vi "LoopScript_EllipticOscillatory.vi"() -> ()   [LabVIEW 2017]
uses:
  CircleControls.ctl
  ImageAcquisitionProgram/ImageAcquisitionLibrary/GlobalFrontPanelReferences.vi
  AODControl/AODGlobals.vi
  AODControl/MessageQueue/QueueOperations/Enqueue Message (Single).vi
  ImageAcquisitionProgram/ImageAcquisitionLibrary/ImageAcquisitionLibrary.lvlib
  AODControl/AODControl.lvlib
  AODControl/MessageQueue/MessageQueue.lvlib
panel:
  in  "Run":bool
  out "Area":dbl
  out "Eccentricity":dbl
  out "Radius":dbl
  in  "Transform\nSeconds":i32=60
  in  "oscillation \nangle":dbl=0.03 format="%#_13g"
  in  "No. of Points":i32=33
  out "Total Running \nTime":dbl=90000.0 format="%<%H:%M:%S>t"
  in  "period (s)":dbl=1.0
  out "Area":dbl[](array[numeric])=[98.5203456165759, 93.52521329736813, 88.53008097816036, 83.5349486589526, 78.53981633974483]
  out "Radius":dbl[](array[numeric])=[5.6, 5.4561891462814955, 5.308483775994799, 5.156549233741495, 5.0]
  out "Eccentricity":dbl[](array[numeric])=[1.0, 1.25, 1.5, 1.75, 2.0]
  in  "e_0":dbl=1.0
  in  "e_f":dbl=2.0
  in  "Eccentricity \nSteps":i32=5
  in  "R_f":dbl=5.0
  in  "R_0":dbl=5.6
  in  "Packing Steps":i32=5
  in  "Number of \nPeriods":u32=3600
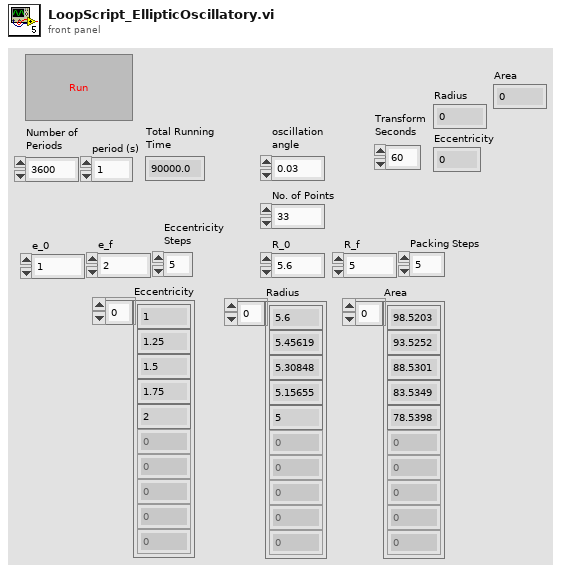
[diagram p1: front panel]
types:
  T1 = typedef "CircleControls.ctl" = cluster{"Radius":dbl, "No. of Points":i32, "Center":cluster{"X":dbl, "Y":dbl}, "Circle":bool, "Density":dbl, "PointSpec":enum32{"No. Of Points", "Density"}, "Hold":bool, "Size":i32, "LatC":dbl, "Eccentricity":dbl, "Phase":dbl}
  T2 = typedef "AODControl.lvlib/InterfaceReferences.ctl" = cluster{"AOD Points Display":refnum<vi>, "AOD Array":refnum<vi>, "AOD Array Size":refnum<vi>, "Replace Array List":refnum<vi>, "Replace List":refnum<vi>, "Remove":refnum<vi>, "Index":refnum<vi>, "Move":refnum<vi>, "X":refnum<vi>, "Y":refnum<vi>, "Add":refnum<vi>, "Load":refnum<vi>, "Save":refnum<vi>, "Exit":refnum<vi>, "Dynamic":refnum<vi>, "Rotate":refnum<vi>, "Rotation Speed":refnum<vi>, "Scaling Speed":refnum<vi>, "X Trans Speed":refnum<vi>, "Y Trans Speed":refnum<vi>, "Movie Array":refnum<vi>, "Play":refnum<vi>, "Playing Time":refnum<vi>}
  T3 = typedef "AODControl.lvlib/MessageQueue.lvlib/All Message Queues.ctl" = cluster{" AOD Interface":refnum<queue>}
  T4 = typedef "ImageAcquisitionLibrary.lvlib/References.ctl" = cluster{"Acquire":refnum<vi>, "Rec":refnum<vi>, "Tracking":refnum<vi>, "Settings":refnum<vi>, "Stop":refnum<vi>, "Initialized?":bool, "ImDisplay":refnum<vi>}
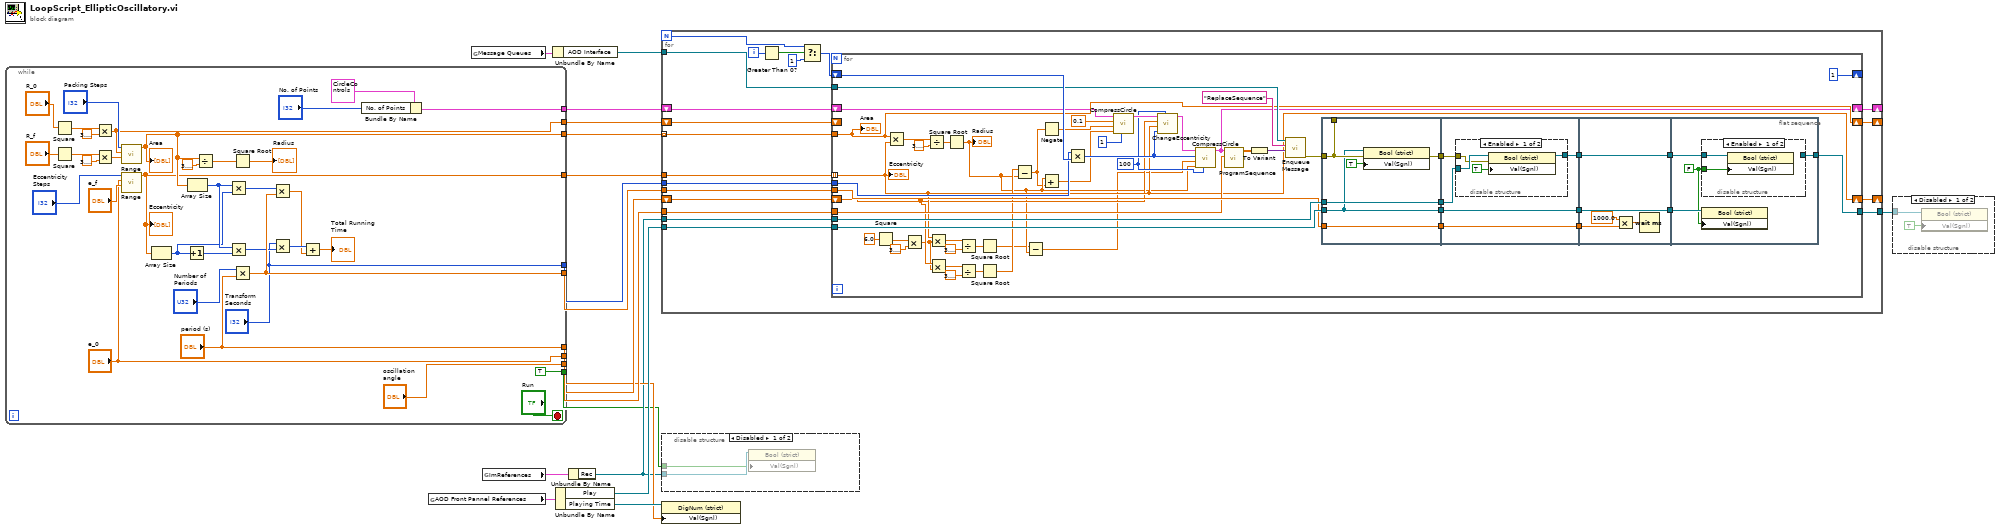
[diagram p0: block diagram]
diagram:
  n1 = while {
    tunnel: [w43] -> w18
    tunnel: [w39] -> w17
    tunnel: ["oscillation \nangle"] -> w16
    tunnel: [w35] -> w12
    tunnel: ["e_0"] -> w11
    tunnel: [w31] -> w10
    tunnel: [w30] -> w7
    tunnel: ["period (s)"] -> w5
    tunnel: ["Transform\nSeconds"] -> w4
    tunnel: [TRUE ("Value (Signaling)")] -> w1
    stop <- "Run" stop-if-true
    n2 = Square(x="R_0") -> (x^2=w51:dbl)
    n3 = Square(x="R_f") -> (x^2=w33:dbl)
    n4 = Multiply(x=w51, y=3.141592653589793) -> (x*y=w31:dbl)
    n5 = Multiply(x=w33, y=3.141592653589793) -> (x*y=w34:dbl)
    n6 = call "Range.vi"("End"=w34, "Start"=w31, "Steps"="Packing Steps") -> ("Array"=w43:dbl[])  [unwired: 8 in]
    "Area" <- w43
    n7 = call "Range.vi"("End"="e_f", "Start"="e_0", "Steps"="Eccentricity \nSteps") -> ("Array"=w35:dbl[])  [unwired: 8 in]
    "Eccentricity" <- w35
    n8 = Array Size(array=w35) -> (size(s)=w27:i32)
    n9 = Array Size(array=w43) -> (size(s)=w28:i32)
    n10 = Increment(x=w27) -> (x+1=w26:i32)
    n11 = Divide(x=w43, y=3.141592653589793) -> (x/y=w46:dbl[])
    n12 = Multiply(x=w28, y=w27) -> (x*y=w42:i32)
    n13 = Multiply(x=w28, y=w26) -> (x*y=w25:i32)
    n14 = Square Root(x=w46) -> (sqrt(x)=→"Radius":dbl[])
    n15 = Multiply(x="Number of \nPeriods", y="period (s)") -> (x*y=w30:dbl)
    n16 = Multiply(x=w42, y=w30) -> (x*y=w22:dbl)
    n17 = Multiply(x="Transform\nSeconds", y=w25) -> (x*y=w23:i32)
    n18 = Add(x=w23, y=w22) -> (x+y=→"Total Running \nTime":dbl)
    n19 = Bundle By Name(cluster=T1 {"Radius"=5.2, "No. of Points"=33, "Center"={"X"=0.0, "Y"=0.0}, "Circle"=TRUE, "Density"=1.0100217542370282, "PointSpec"=enum."No. Of Points", "Hold"=FALSE, "Size"=1, "LatC"=10.0, "Eccentricity"=1.0, "Phase"=0.0} ("Cluster"), "No. of Points"="No. of Points") -> (w39:T1)
  }
  n20 = global read "AODGlobals.vi" "AOD Front Pannel References"() -> (w9:T2)
  n21 = global read "AODGlobals.vi" "Message Queues"() -> (w14:T3)
  n22 = global read "GlobalFrontPanelReferences.vi" "ImReferences"() -> (w15:T4)
  n23 = Unbundle By Name(w14) -> ("AOD Interface"=w13:refnum<queue>)
  n24 = Unbundle By Name(w9) -> ("Play"=w8:refnum<vi>, "Playing Time"=w6:refnum<vi>)
  n25 = Unbundle By Name(w15) -> ("Rec"=w3:refnum<vi>)
  n26 = for {
    N -> [w58]
    tunnel: w18 -> [w67] mode=indexing
    tunnel: w12 -> [w56]
    tunnel: w16 -> [w73]
    tunnel: w13 -> [w72]
    tunnel: w4 -> [w71]
    shift-right: [w68] -> _
    shift-left: w10 -> [w66]
    shift-right: [w70] -> _
    shift-left: w11 -> [w69]
    tunnel: w8 -> [w65]
    tunnel: w3 -> [w64]
    tunnel: w7 -> [w63]
    tunnel: [w62] -> w2
    shift-right: [w55] -> _
    shift-left: w17 -> [w54]
    i -> [w61]
    n27 = Greater Than 0?(x=w61) -> (x > 0?=w60:bool)
    n28 = Select(t=w58, s=w60, f=1) -> (s? t:f=w57:i32)
    n29 = for {
      tunnel: w56 -> [w87] mode=indexing
      tunnel: w67 -> [w105]
      tunnel: w73 -> [w103]
      shift-right: [w105] -> w68
      shift-left: w66 -> [_]
      tunnel: w72 -> [w106]
      tunnel: w71 -> [w104]
      shift-right: [w87] -> w70
      shift-left: w69 -> [w80]
      tunnel: w65 -> [w122]
      tunnel: w64 -> [w119]
      tunnel: w63 -> [w116]
      shift-right: [1] -> _
      shift-left: w57 -> [w112]
      tunnel: [w107] -> w62
      shift-right: [w92] -> w55
      shift-left: w54 -> [w91]
      w97 = 100 ("Steps")
      n30 = Square(x=6.0 ("Delta R")) -> (x^2=w88:dbl)
      n31 = Multiply(x=w105, y=w87) -> (x*y=w100:dbl)
      n32 = Multiply(x=w88, y=3.141592653589793) -> (x*y=w79:dbl)
      n33 = Divide(x=w100, y=3.141592653589793) -> (x/y=w101:dbl)
      n34 = Multiply(x=w87, y=w79) -> (x*y=w86:dbl)
      n35 = Multiply(x=w80, y=w79) -> (x*y=w81:dbl)
      n36 = Square Root(x=w101) -> (sqrt(x)=w77:dbl)
      "Radius" <- w77
      n37 = Divide(x=w86, y=3.141592653589793) -> (x/y=w84:dbl)
      n38 = Divide(x=w81, y=3.141592653589793) -> (x/y=w83:dbl)
      n39 = Square Root(x=w84) -> (sqrt(x)=w76:dbl)
      n40 = Square Root(x=w83) -> (sqrt(x)=w78:dbl)
      n41 = Subtract(x=w78, y=w77) -> (x-y=w75:dbl)
      n42 = Subtract(x=w76, y=w77) -> (x-y=w74:dbl)
      n43 = Negate(x=w75) -> (-x=w96:dbl)
      n44 = Add(x=w77, y=w75) -> (x+y=w93:dbl)
      n45 = Multiply(x=w104, y=w112) -> (x*y=w98:i32)
      n46 = call "CompressCircle.vi"("Steps"=u32 1, "R0"=w93, "Delta R"=w96, "Time"=0.1, "input ellipse params"=w91) -> ("output ellipse params"=w102:T1)  [unwired: 5 in, 1 out]
      n47 = call "ChangeEccentricity.vi"("Steps"=w97, "Time"=w98, "e_f"=w87, "e_0"=w80, "Cluster in"=w102) -> ("Cluster out"=w99:T1)  [unwired: 6 in]
      n48 = call "CompressCircle.vi"("Steps"=w97, "R0"=w77, "Delta R"=w74, "Time"=w98, "input ellipse params"=w99) -> ("output ellipse params"=w92:T1)  [unwired: 5 in, 1 out]
      n49 = call "ProgramSequence.vi"("Angle"=w103, "Cluster"=w92) -> ("Sequence"=w124:dbl[][][])  [unwired: 9 in]
      n50 = To Variant(anything=w124) -> (Variant=w125:variant)
      n51 = call-poly "Enqueue Message.vi"("Message Data"=w125, "Message"="ReplaceSequence", "Message Queue"=w106) -> ("error out"=w121:errorcluster)  [unwired: 7 in, 1 out]
      n52 = flat-sequence {
        tunnel: w122 -> [w127]
        tunnel: [w131] -> _
        tunnel: w121 -> [w131]
        tunnel: [w130] -> w120
        tunnel: w119 -> [w130]
        tunnel: [w129] -> w118
        tunnel: [w128] -> w117
        tunnel: w116 -> [w128]
        tunnel: [w127] -> w110
        tunnel: w120 -> [w137]
        tunnel: w118 -> [w136]
        tunnel: w117 -> [w135]
        tunnel: [w135] -> w115
        tunnel: [w134] -> w113
        tunnel: w110 -> [w133]
        tunnel: [w133] -> w109
        tunnel: w115 -> [w146]
        tunnel: [w143] -> w114
        tunnel: w113 -> [w143]
        tunnel: w109 -> [w142]
        tunnel: [w142] -> w108
        tunnel: w114 -> [w150]
        tunnel: w108 -> [w149]
        tunnel: [w147] -> w107
        frame #0 {
          n53 = property class="Bool (strict)"(reference=w127, error in=w131, "Val(Sgnl)"=TRUE ("Value (Signaling)")) -> (error out=w129:errorcluster)  [unwired: 1 out]
        }
        frame #1 {
          n54 = disable-structure shown="Enabled" {
            disable-tunnel: w137 -> [w141 _]
            disable-tunnel: w136 -> [w139 _]
            disable-tunnel: [w138 _] -> w134
            frame Enabled {
              n55 = property class="Bool (strict)"(reference=w141, error in=w139, "Val(Sgnl)"=TRUE ("Value (Signaling)")) -> (reference out=w138:refnum<vi>)  [unwired: 1 out]
            }
            frame Disabled {
            }
          }
        }
        frame #2 {
          n56 = Multiply(x=1000.0, y=w146) -> (x*y=w144:dbl)
          n57 = Wait (ms)(milliseconds to wait=w144) -> ()  [unwired: 1 out]
        }
        frame #3 {
          w148 = FALSE ("Value (Signaling)")
          n58 = disable-structure shown="Enabled" {
            disable-tunnel: w150 -> [w152 w153]
            disable-tunnel: w148 -> [w151 _]
            disable-tunnel: [_ w153] -> w147
            frame Enabled {
              n59 = property class="Bool (strict)"(reference=w152, "Val(Sgnl)"=w151) -> ()  [unwired: 1 in, 2 out]
            }
            frame Disabled {
            }
          }
          n60 = property class="Bool (strict)"(reference=w149, "Val(Sgnl)"=w148) -> ()  [unwired: 1 in, 2 out]
        }
      }
      "Eccentricity" <- w87
      "Area" <- w105
    }
  }
  n61 = disable-structure shown="Disabled" {
    disable-tunnel: w3 -> [w155 _]
    disable-tunnel: w1 -> [w154 _]
    frame Disabled {
      n62 = property class="Bool (strict)"(reference=w155, "Val(Sgnl)"=w154) -> ()  [unwired: 1 in, 2 out]
    }
    frame Enabled {
    }
  }
  n63 = property class="DigNum (strict)"(reference=w6, "Val(Sgnl)"=w5) -> ()  [unwired: 1 in, 2 out]
  n64 = disable-structure shown="Disabled" {
    disable-tunnel: w2 -> [w156 _]
    frame Disabled {
      n65 = property class="Bool (strict)"(reference=w156, "Val(Sgnl)"=TRUE ("Value (Signaling)")) -> ()  [unwired: 1 in, 2 out]
    }
    frame Enabled {
    }
  }
